vi "convert_spreadsheet_to_graph.vi"(9 "all rows":dbl[][](array[numeric])) -> (3 "Array":cluster{dbl[], dbl[]}[](array[cluster]))   [LabVIEW 2015]
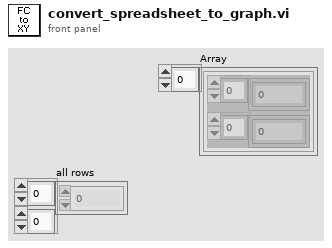
[diagram p1: front panel]
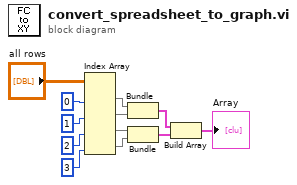
[diagram p0: block diagram]
diagram:
  n1 = Index Array(array="all rows", index (col) #1=0 ("disabled index (col)"), index (col) #2=1 ("index (col)"), index (col) #3=2 ("index (col)"), index (col) #4=3 ("index (col)")) -> (element #1=w4:dbl[], element #2=w3:dbl[], element #3=w2:dbl[], element #4=w1:dbl[])  [unwired: 4 in]
  n2 = Bundle("all rows"=w4, "all rows"=w3) -> (w6:cluster{"all rows":dbl[], "all rows":dbl[]})  [unwired: 1 in]
  n3 = Bundle("all rows"=w2, "all rows"=w1) -> (w5:cluster{"all rows":dbl[], "all rows":dbl[]})  [unwired: 1 in]
  n4 = Build Array(w6, w5) -> (→"Array":cluster{"all rows":dbl[], "all rows":dbl[]}[])
